vi "Write to Text File and Read from Text File.vi"() -> ()   [LabVIEW 2023]
doc: "This example shows how the Write to Text File and Read from Text File functions operate using different options."
panel:
  out "Read Text (multiple lines)":string[](array[string])
  in  "Read Count (multiple lines)":i32=-1
  out "Read Text":string="\n"
  in  "Write Text":string="Line 1 of Text File.\nLine 2 of Text File.\nLine 3 of Text File."
  in  "Operation":u16(ring) items=["Input File as Path", "Input File as Refnum", "Deselecting Convert EOL", "Specifying Read Lines (single line)", "Specifying Read Lines (multiple lines)"]
  # "Overview: Demonstrates the use of the Write to Text File function to write data to a text file, and the Read from Text File function to read data from that text file.\nInstructions:\n1. Specify an Operation to illustrate a particular use case for the Write to Text File and Read from Text File functions.\n2. Run the VI. The 'Write' values below will be written to the file, then read back and displayed in the 'Read' values.\n3. Delete the text file (located at [LabVIEW Data]\\Example Write Read Text File.txt) when you are done."
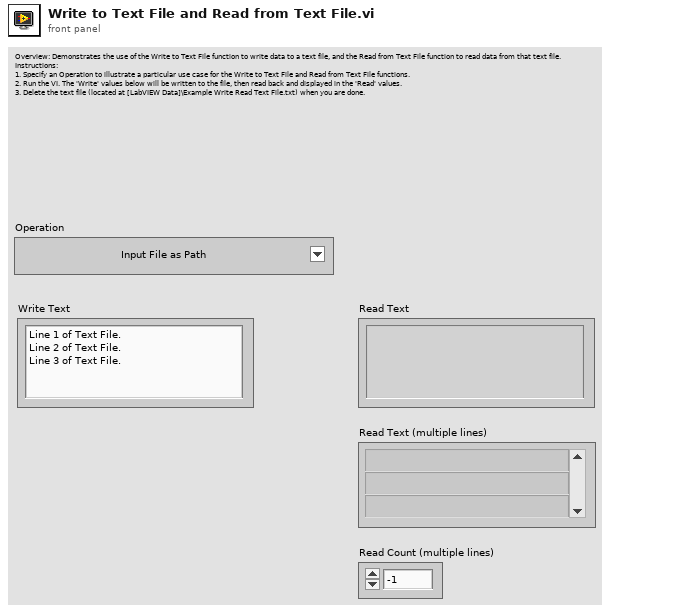
[diagram p1: front panel]
types:
  T1 = enum16{"open", "replace", "create", "open or create", "replace or create", "replace or create with confirmation"}
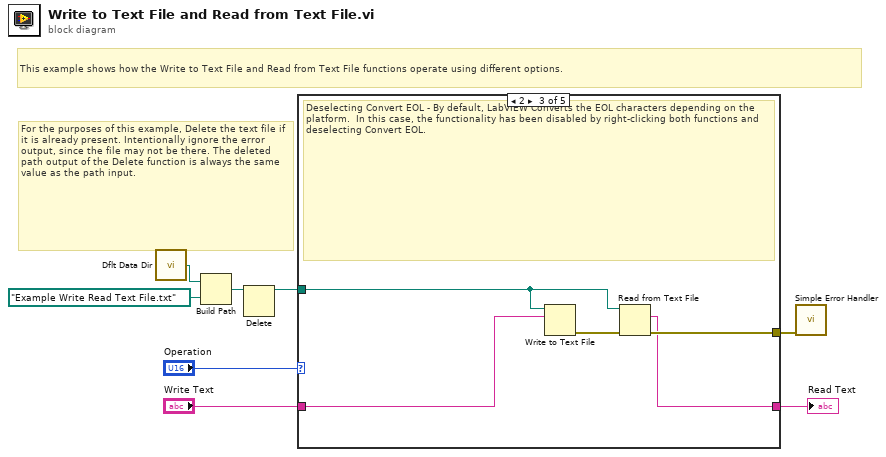
[diagram p0: block diagram]
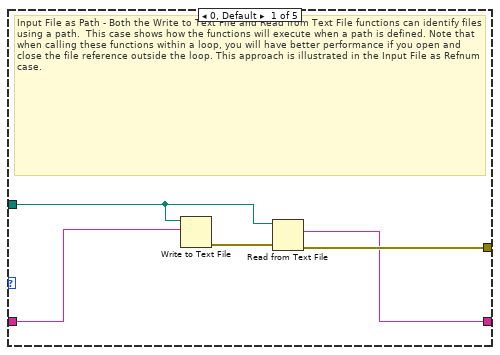
[diagram p2: hidden frame]
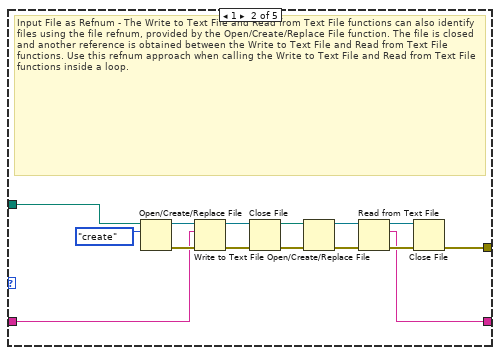
[diagram p3: hidden frame]
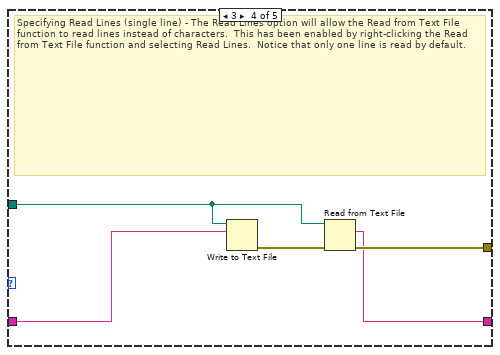
[diagram p4: hidden frame]
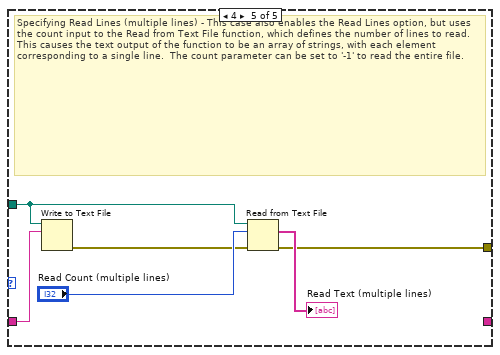
[diagram p5: hidden frame]
diagram:
  # "This example shows how the Write to Text File and Read from Text File functions operate using different options."
  # "For the purposes of this example, Delete the text file if it is already present. Intentionally ignore the error output, since the file may not be there. The deleted path output of the Delete function is always the same value as the path input."
  n1 = call <vilib>:"Dflt Data Dir.vi"() -> ("App:Default Data Directory"=w6:path)
  n2 = Build Path(base path=w6, name or relative path=path "Example Write Read Text File.txt" ("default name")) -> (appended path=w4:path)
  n3 = Delete(path (use dialog)=w4) -> (deleted path=w3:path)  [unwired: 4 in, 2 out]
  n4 = case shown="2" "Operation" {
    tunnel: [w12 w23 w32 w37 w41] -> w1
    tunnel: "Write Text" -> [w11 w16 w31 w36 w40]
    tunnel: [w10 w15 w30 w35 _] -> w7
    tunnel: w3 -> [w9 w14 w29 w34 w39]
    frame 0, Default {
      # "Input File as Path - Both the Write to Text File and Read from Text File functions can identify files using a path.  This case shows how the functions will execute when a path is defined. Note that when calling these functions within a loop, you will have better performance if you open and close the file reference outside the loop. This approach is illustrated in the Input File as Refnum case."
      n5 = Write to Text File(file (use dialog)=w9, text=w11) -> (error out=w13:errorcluster)  [unwired: 2 in, 2 out]
      n6 = Read from Text File(file (use dialog)=w9, error in=w13) -> (text=w10:string, error out=w12:errorcluster)  [unwired: 2 in, 2 out]
    }
    frame 1 {
      # "Input File as Refnum - The Write to Text File and Read from Text File functions can also identify files using the file refnum, provided by the Open/Create/Replace File function. The file is closed and another reference is obtained between the Write to Text File and Read from Text File functions. Use this refnum approach when calling the Write to Text File and Read from Text File functions inside a loop."
      n7 = Open/Create/Replace File(file path (use dialog)=w14, operation (0:open)=T1."create") -> (refnum out=w26:refnum<file>, error out=w28:errorcluster)  [unwired: 4 in, 1 out]
      n8 = Write to Text File(file (use dialog)=w26, text=w16, error in=w28) -> (refnum out=w22:refnum<file>, error out=w18:errorcluster)  [unwired: 1 in, 1 out]
      n9 = Close File(refnum=w22, error in=w18) -> (path=w21:path, error out=w20:errorcluster)
      n10 = Open/Create/Replace File(file path (use dialog)=w21, error in=w20) -> (refnum out=w19:refnum<file>, error out=w17:errorcluster)  [unwired: 4 in, 1 out]
      n11 = Read from Text File(file (use dialog)=w19, error in=w17) -> (refnum out=w25:refnum<file>, text=w15:string, error out=w24:errorcluster)  [unwired: 2 in, 1 out]
      n12 = Close File(refnum=w25, error in=w24) -> (error out=w23:errorcluster)  [unwired: 1 out]
    }
    frame 2 {
      # "Deselecting Convert EOL - By default, LabVIEW Converts the EOL characters depending on the platform.  In this case, the functionality has been disabled by right-clicking both functions and deselecting Convert EOL."
      n13 = Write to Text File(file (use dialog)=w29, text=w31) -> (error out=w33:errorcluster)  [unwired: 2 in, 2 out]
      n14 = Read from Text File(file (use dialog)=w29, error in=w33) -> (text=w30:string, error out=w32:errorcluster)  [unwired: 2 in, 2 out]
    }
    frame 3 {
      # "Specifying Read Lines (single line) - The Read Lines option will allow the Read from Text File function to read lines instead of characters.  This has been enabled by right-clicking the Read from Text File function and selecting Read Lines.  Notice that only one line is read by default."
      n15 = Write to Text File(file (use dialog)=w34, text=w36) -> (error out=w38:errorcluster)  [unwired: 2 in, 2 out]
      n16 = Read from Text File(file (use dialog)=w34, error in=w38) -> (text=w35:string, error out=w37:errorcluster)  [unwired: 2 in, 2 out]
    }
    frame 4 {
      # "Specifying Read Lines (multiple lines) - This case also enables the Read Lines option, but uses the count input to the Read from Text File function, which defines the number of lines to read. This causes the text output of the function to be an array of strings, with each element corresponding to a single line.  The count parameter can be set to '-1' to read the entire file."
      n17 = Write to Text File(file (use dialog)=w39, text=w40) -> (error out=w42:errorcluster)  [unwired: 2 in, 2 out]
      n18 = Read from Text File(file (use dialog)=w39, count="Read Count (multiple lines)", error in=w42) -> (text=→"Read Text (multiple lines)":string[], error out=w41:errorcluster)  [unwired: 1 in, 2 out]
    }
  }
  "Read Text" <- w7
  n19 = call <vilib>:"Simple Error Handler.vi"("error in (no error)"=w1) -> ()  [unwired: 4 in, 5 out]
